vi "CRYGet Excel Header.vi"(7 "Type":enum16{"Curves", "Values", "Results", "WFM"}(ring), 9 "Waveform":T1={"Waveform"={"X0"=0.0, "dX"=0.0, "Y"=[]}, "X data"=1, "Y data"=1, "Y axis"=1, "X unit"="s", "Y unit"="V", "Y dB ref"=1.0, "display Y"=TRUE, "display X"=TRUE, "Overload?"=FALSE, "Test Info"="", "Step No."=0, "Name"="", "protected"=FALSE, "Sqc history"=[], "Signal Channel ID"=0, "Plot Settings"={"Color"=0, "Interpolation"=0, "Point Style"=0, "Line Style"=0, "Point Color"=0, "Line Width"=0, "Bar Plot Style"=0, "Fill To"=0}, "AutoProtect"=FALSE} {"Y dB ref" format="%.1f"; "Y axis" items=["Log", "Lin"]; "Y data" items=["dB", "Lin"]; "X data" items=["dB", "Lin"]}, 10 "Curve":T2={"Name"="", "Curve"=[], "X data"=1, "Y data"=1, "Z data"=1, "X axis"=0, "Y axis"=1, "Z axis"=1, "X unit"="Hz", "Y unit"="", "Z unit"="deg.", "X dB ref"=1.0, "Y dB ref"=1.0, "Z dB ref"=1.0, "single val"=FALSE, "protected"=FALSE, "display X"=TRUE, "display Y"=TRUE, "display Z"=TRUE, "Test Info"="", "Step No."=0, "Plot Settings"={"Color"=0, "Interpolation"=0, "Point Style"=0, "Line Style"=0, "Point Color"=0, "Line Width"=0, "Bar Plot Style"=0, "Fill To"=0}, "AutoProtect"=FALSE} {"Z data" items=["dB", "Lin"]; "X data" items=["dB", "Lin"]; "Y data" items=["dB", "Lin"]; "Z dB ref" format="%.1f"; "Z axis" items=["Log", "Lin"]; "X dB ref" format="%.1f"; "X axis" items=["Log", "Lin"]; "Y axis" items=["Log", "Lin"]; "Y dB ref" format="%.1f"; "Curve"."z" format="%.2f"; "Curve"."y" format="%.2f"; "Curve"."x" format="%.2f"}, 11 "Export format":T3) -> (3 "Header String":string[][](array[string]))   [LabVIEW 2013]
uses:
  CRYSystem/Typedef Control/CRYData Cluster.ctl
  CRYSystem/Typedef Control/CRYWaveform Cluster.ctl
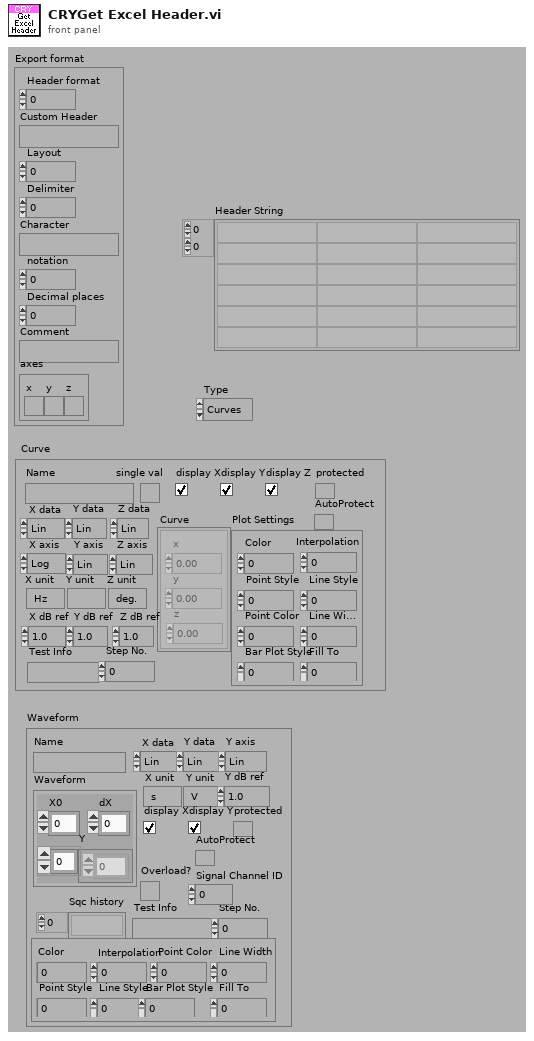
[diagram p1: front panel]
types:
  T1 = typedef "CRYWaveform Cluster.ctl" = cluster{"Waveform":cluster{"X0":dbl, "dX":dbl, "Y":sgl[]}, "X data":u16, "Y data":u16, "Y axis":u16, "X unit":string, "Y unit":string, "Y dB ref":dbl, "display Y":bool, "display X":bool, "Overload?":bool, "Test Info":string, "Step No.":i32, "Name":string, "protected":bool, "Sqc history":string[], "Signal Channel ID":i32, "Plot Settings":cluster{"Color":u32, "Interpolation":u8, "Point Style":u8, "Line Style":u8, "Point Color":u32, "Line Width":u8, "Bar Plot Style":u8, "Fill To":i16}, "AutoProtect":bool}
  T2 = typedef "CRYData Cluster.ctl" = cluster{"Name":string, "Curve":cluster{"x":dbl, "y":dbl, "z":dbl}[], "X data":u16, "Y data":u16, "Z data":u16, "X axis":u16, "Y axis":u16, "Z axis":u16, "X unit":string, "Y unit":string, "Z unit":string, "X dB ref":dbl, "Y dB ref":dbl, "Z dB ref":dbl, "single val":bool, "protected":bool, "display X":bool, "display Y":bool, "display Z":bool, "Test Info":string, "Step No.":i32, "Plot Settings":cluster{"Color":u32, "Interpolation":u8, "Point Style":u8, "Line Style":u8, "Point Color":u32, "Line Width":u8, "Bar Plot Style":u8, "Fill To":i16}, "AutoProtect":bool}
  T3 = cluster{"Header format":u16, "Custom Header":string, "Layout":u16, "Delimiter":i32, "Character":string, "notation":u16, "Decimal places":i32, "Comment":string, "axes":cluster{"x":bool, "y":bool, "z":bool}}
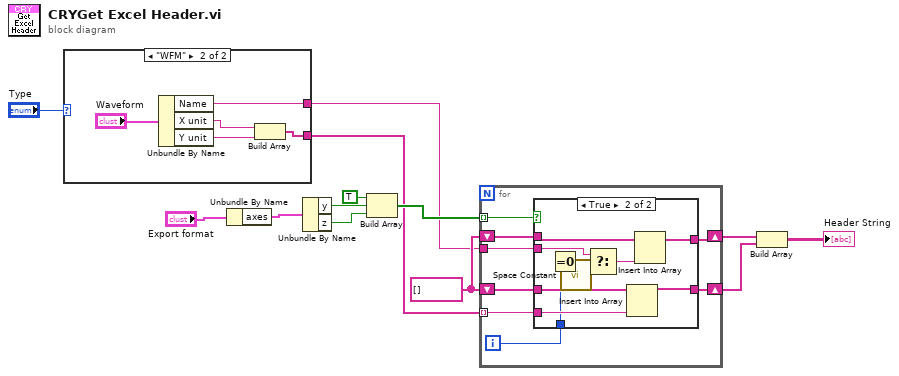
[diagram p0: block diagram]
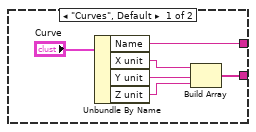
[diagram p2: hidden frame]
diagram:
  w8 = string[] [] ("appended array")
  n1 = case shown="\"WFM\"" "Type" {
    tunnel: [w19 w24] -> w9
    tunnel: [w14 w21] -> w4
    frame "Curves", Default {
      n2 = Unbundle By Name("Curve") -> ("Name"=w14:string, "X unit"=w17:string, "Y unit"=w16:string, "Z unit"=w15:string)
      n3 = Build Array(w17, w16, w15) -> (w19:string[])
    }
    frame "WFM" {
      n4 = Unbundle By Name("Waveform") -> ("Name"=w21:string, "X unit"=w23:string, "Y unit"=w22:string)
      n5 = Build Array(w23, w22) -> (w24:string[])
    }
  }
  n6 = Unbundle By Name("Export format") -> ("axes"=w5:cluster{"x":bool, "y":bool, "z":bool})
  n7 = Unbundle By Name(w5) -> ("y"=w13:bool, "z"=w12:bool)
  n8 = Build Array(TRUE ("element"), w13, w12) -> (w11:bool[])
  n9 = for {
    tunnel: w11 -> [w32] mode=indexing
    tunnel: w9 -> [w29] mode=indexing
    shift-right: [w30] -> w7
    shift-left: w8 -> [w31]
    tunnel: w4 -> [w25]
    shift-right: [w26] -> w3
    shift-left: w8 -> [w27]
    i -> [w28]
    n10 = case shown="True" w32 {
      tunnel: w31 -> [w34 w44]
      tunnel: [w34 w43] -> w30
      tunnel: w29 -> [_ w42]
      tunnel: w28 -> [_ w39]
      tunnel: w27 -> [w33 w38]
      tunnel: [w33 w37] -> w26
      tunnel: w25 -> [_ w36]
      frame False {
      }
      frame True {
        n11 = Equal To 0?(x=w39) -> (x = 0?=w40:bool)
        n12 = call <vilib>:"Space Constant.vi"() -> ("String"=w35:string)
        n13 = Select(t=w36, s=w40, f=w35) -> (s? t:f=w41:string)
        n14 = Insert Into Array(array=w44, new element=w42) -> (w43:string[])  [unwired: 1 in]
        n15 = Insert Into Array(array=w38, new element=w41) -> (w37:string[])  [unwired: 1 in]
      }
    }
  }
  n16 = Build Array(w3, w7) -> (→"Header String":string[][])
